vi "cluster_v05.vi"() -> ()   [LabVIEW 2009]
panel:
  in  "stop":bool
  in  "n":dbl(slide)=4.716312056737589 scale=0.0..10.0
  out "XY Graph- Roza polara":cluster{dbl[], dbl[]}(graph)={[0.8863779204775526, 0.20767050007480056, 0.4479177124922344, 0.46439069249595577, -0.5079083010395595, 0.17830171218080154, -0.8651661995665252, -0.3276439863376904, -0.21337700033403872, -0.4601220595212925, 0.6809078808366298, -0.051320374794149186, 0.7757141046304956, 0.42976166282399564, -0.03212505394145438, 0.41528640042491305, -0.7952848094330506, -0.09116223500951781, -0.6269883936271136, -0.5032133784530356, 0.26844548135391805, -0.33066802749575647, 0.8433272239305906, 0.23744706721762524, 0.43260813457059466, 0.5390972050562264, -0.47671286005255337, 0.21083299306886094, -0.8229855511073545, -0.37465479822704834, -0.20959111687240997, -0.531387517318898, 0.6408751528809078, -0.06392628661170396, 0.7379005904304059, 0.4898760514311481, -0.023159142938157882, 0.47767685045444697, -0.7489709107006614, -0.09888459409041829, -0.5969468838313164, -0.5713832392338134, 0.24648963447078878, -0.3796102607441805, 0.7940204105863203, 0.2642814246475509, 0.4133418249753996, 0.6097904504231993, -0.44261319390008297, 0.24295759009333803, -0.7744686563848888, -0.4179124523369327, -0.2034078576673542, -0.5990487442303393, 0.5965637318515186, -0.07730175040383354, 0.6941528687318052, 0.5456591725252956, -0.014896424536584397, 0.5371759569097828, -0.6973692613257292, -0.10464308414277707, -0.5618094092076609], [0.0889344379948988, 0.4080226205476214, -0.765870552210542, -0.01932638704238845, -0.7230209175640688, -0.4367303265962668, 0.16028262004853602, -0.34890582911567924, 0.8497521920283285, 0.15492333966419736, 0.5452637472598225, 0.4896657433507465, -0.39050100067210575, 0.25390438207859417, -0.863946810348284, -0.28899428326212423, -0.32880078943302865, -0.5045274950892685, 0.5835803075586783, -0.12872953395643427, 0.8091059487237997, 0.40920262706177457, 0.09216165433696126, 0.4769225580271859, -0.7248929887578119, -0.01765701471275406, -0.6915469631331344, -0.5036266737651522, 0.14494566086310778, -0.4061116710916178, 0.8044621189419148, 0.17369711782872047, 0.5225830044698135, 0.5619194312457269, -0.3633147875692448, 0.29530064307210513, -0.8176772393176024, -0.32617387367966444, -0.31744422842398284, -0.5763772180888083, 0.5458376189294349, -0.15156930675919417, 0.7655358790316874, 0.46135494204667443, 0.09389246023124602, 0.5428104250354701, -0.6788816752244404, -0.014570546267764018, -0.6544008728940885, -0.5662408269994127, 0.1293438069690215, -0.46112498422749076, 0.7533343525358808, 0.18996165376249866, 0.49530615527626576, 0.6298038546706766, -0.3341742283630108, 0.33554750575981246, -0.7652318826519705, -0.3598718339388323, -0.3028825524162445, -0.6441004817700923, 0.5046510499842722]}
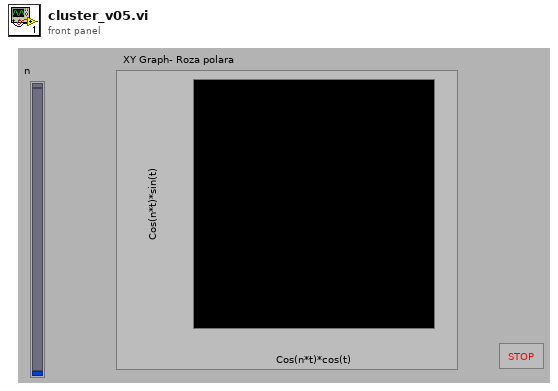
[diagram p1: front panel]
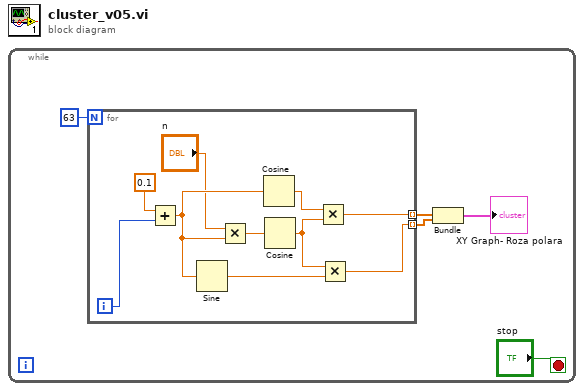
[diagram p0: block diagram]
diagram:
  n1 = while {
    stop <- "stop" stop-if-true
    n2 = for {
      N: 63 -> [_]
      tunnel: [w11] -> w4 mode=indexing
      tunnel: [w7] -> w3 mode=indexing
      i -> [w15]
      n3 = Add(x=0.1, y=w15) -> (x+y=w10:dbl)
      n4 = Sine(x=w10) -> (sin(x)=w8:dbl)
      n5 = Multiply(x="n", y=w10) -> (x*y=w13:dbl)
      n6 = Cosine(x=w10) -> (cos(x)=w12:dbl)
      n7 = Cosine(x=w13) -> (cos(x)=w9:dbl)
      n8 = Multiply(x=w12, y=w9) -> (x*y=w11:dbl)
      n9 = Multiply(x=w9, y=w8) -> (x*y=w7:dbl)
    }
    n10 = Bundle(w4, w3) -> (→"XY Graph- Roza polara":cluster{dbl[], dbl[]})  [unwired: 1 in]
  }
